vi "CC_CreateNewCTL.vi"(8 "Error In":errorcluster, 9 "Settings":T1, 10 "Save Path":path, 11 "Clipboard Data":string[][](array[string])) -> (0 "Error Out":errorcluster)   [LabVIEW 2014]
uses:
  <vilib>/JDP Science/JDP Science Common Utilities/JDP Utility.lvlib
  controls/CC_AppendMode.ctl
  controls/CC_TypeSelectionEnum.ctl
  controls/CC_CreateNewCTLSettings.ctl
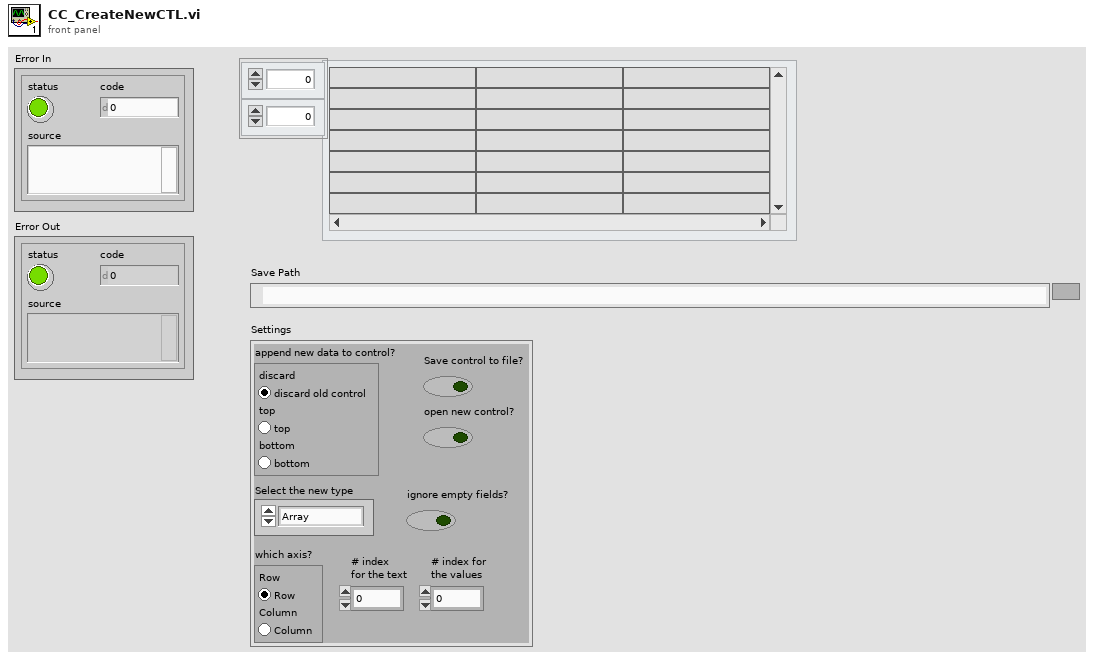
[diagram p1: front panel]
types:
  T1 = typedef "CC_CreateNewCTLSettings.ctl" = cluster{"Save control to file?":bool, "ignore empty fields?":bool, "# index\nfor the text":i32, "# index for\nthe values":i32, "Select the new type":T2, "which axis?":enum32{"Row", "Column"}, "append new data to control?":enum32{"discard", "top", "bottom"}, "open new control?":bool}
  T2 = typedef "CC_TypeSelectionEnum.ctl" = enum16{"Array", "Enum", "Ring", "Text Combobox"}
  T3 = typedef "CC_AppendMode.ctl" = enum16{"discard old control", "top", "bottom"}
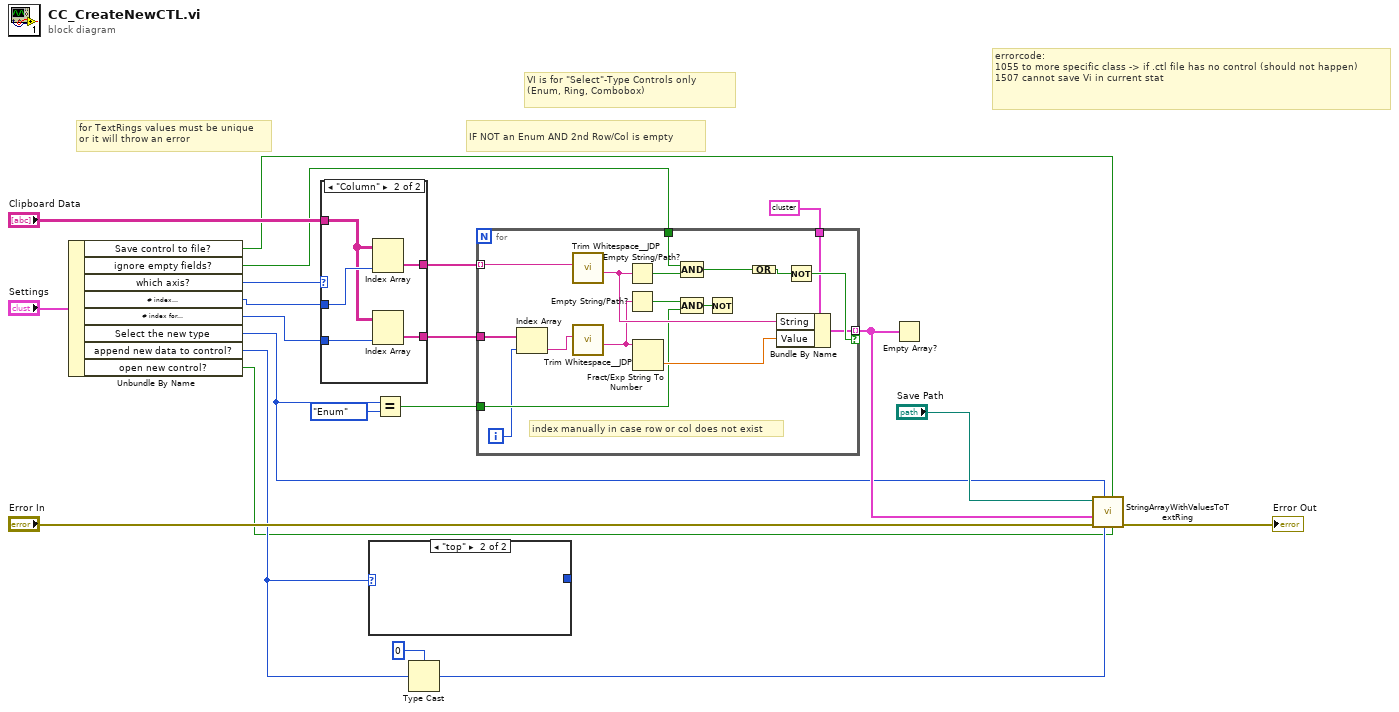
[diagram p0: block diagram]
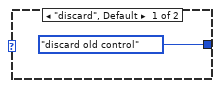
[diagram p2: hidden frame]
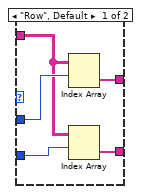
[diagram p3: hidden frame]
diagram:
  # "IF NOT an Enum AND 2nd Row/Col is empty"
  # "VI is for \"Select\"-Type Controls only\n(Enum, Ring, Combobox)"
  # "errorcode: \n1055 to more specific class -> if .ctl file has no control (should not happen)\n1507 cannot save Vi in current stat"
  # "for TextRings values must be unique\nor it will throw an error"
  n1 = Unbundle By Name("Settings") -> ("Save control to file?"=w10:bool, "ignore empty fields?"=w11:bool, "which axis?"=w9:enum32{"Row", "Column"}, "# index\nfor the text"=w8:i32, "# index for\nthe values"=w7:i32, "Select the new type"=w3:T2, "append new data to control?"=w6:enum32{"discard", "top", "bottom"}, "open new control?"=w5:bool)
  n2 = case shown="\"Column\"" w9 {
    tunnel: "Clipboard Data" -> [w24 w28]
    tunnel: [w26 w31] -> w20
    tunnel: w8 -> [w25 w30]
    tunnel: w7 -> [w23 w27]
    tunnel: [w22 w29] -> w19
    frame "Row", Default {
      n3 = Index Array(array=w24, index (row)=w25) -> (element=w26:string[])  [unwired: 1 in]
      n4 = Index Array(array=w24, index (row)=w23) -> (element=w22:string[])  [unwired: 1 in]
    }
    frame "Column" {
      n5 = Index Array(array=w28, index (col)=w30) -> (element=w31:string[])  [unwired: 1 in]
      n6 = Index Array(array=w28, index (col)=w27) -> (element=w29:string[])  [unwired: 1 in]
    }
  }
  n7 = case shown="\"top\"" w6 {
    tunnel: [CC_AppendMode."discard old control" ("append mode") _] -> _
    frame "discard", Default {
    }
    frame "top" {
    }
  }
  n8 = Equal?(x=w3, y=CC_TypeSelectionEnum."Enum") -> (x = y?=w1:bool)
  n9 = Type Cast(type=0, x=w6) -> (*(type *) &x=w16:i32)
  n10 = for {
    tunnel: w20 -> [w49] mode=indexing
    tunnel: w11 -> [w35]
    tunnel: [w44] -> w4 mode=indexing if=w48
    tunnel: w19 -> [w40]
    tunnel: cluster{"String":string, "Value":ext} {"String"="", "Value"=0.0} -> [w47]
    tunnel: w1 -> [w41]
    i -> [w38]
    # "index manually in case row or col does not exist"
    n11 = Index Array(array=w40, index=w38) -> (element=w39:string)
    n12 = call <vilib>:"Trim Whitespace__JDP.vi"("String in"=w49) -> ("String out"=w46:string)  [unwired: 6 in]
    n13 = call <vilib>:"Trim Whitespace__JDP.vi"("String in"=w39) -> ("String out"=w43:string)  [unwired: 6 in]
    n14 = Empty String/Path?(string/path=w46) -> (empty?=w34:bool)
    n15 = Empty String/Path?(string/path=w43) -> (empty?=w42:bool)
    n16 = Fract/Exp String To Number(string=w43) -> (number=w45:dbl)  [unwired: 3 in, 1 out]
    n17 = Compound Arithmetic op=AND(w35, w34) -> (w33:bool)
    n18 = Compound Arithmetic op=AND(w42, w41) -> (w37:bool)
    n19 = Not(x=w37) -> ()  [unwired: 1 out]
    n20 = Compound Arithmetic op=OR(w33) -> (w36:bool)
    n21 = Bundle By Name(cluster=w47, "String"=w46, "Value"=w45) -> (w44:cluster{"String":string, "Value":ext})
    n22 = Not(x=w36) -> (.not. x?=w48:bool)
  }
  n23 = Empty Array?(array=w4) -> ()  [unwired: 1 out]
  n24 = call "StringArrayWithValuesToTextRing.vi"("open new control?"=w5, "auto-Save new Typedef (F)"=w10, "append mode"=w16, "TypeSelection"=w3, "Error In"="Error In", "Strings And Values []"=w4, "Save TypDef Path"="Save Path") -> ("Error Out"=→"Error Out":errorcluster)  [unwired: 4 in]
